vi "Dispose Report.vi"(0 "report in":refnum<class "NI_Word.lvclass">, 5 "wait until printing completed? (T)":bool=TRUE, 9 "save changes? (F)":bool, 11 "error in (no error)":errorcluster, 12 "close report? (T)":bool=TRUE) -> (15 "error out":errorcluster)   [LabVIEW 2015, in "NI_Word.lvclass"]
doc: "Closes the report and releases its interface, which saves memory."
uses:
  <vilib>/Utility/NIReport.llb/Word/NI_Word.lvclass
  <vilib>/Utility/NIReport.llb/Word/NI_Word.lvclass/NI_Word.ctl
  <vilib>/addons/_office/NI_ReportGenerationToolkit.lvlib
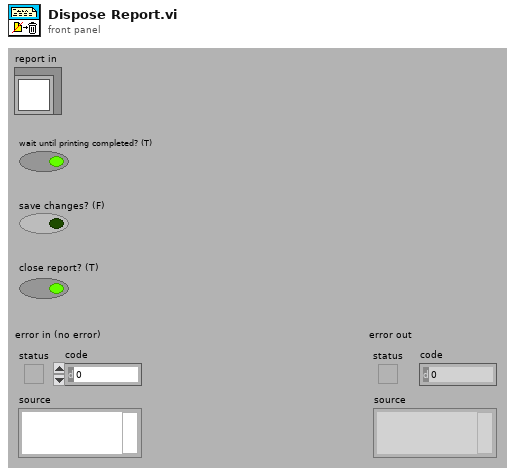
[diagram p1: front panel]
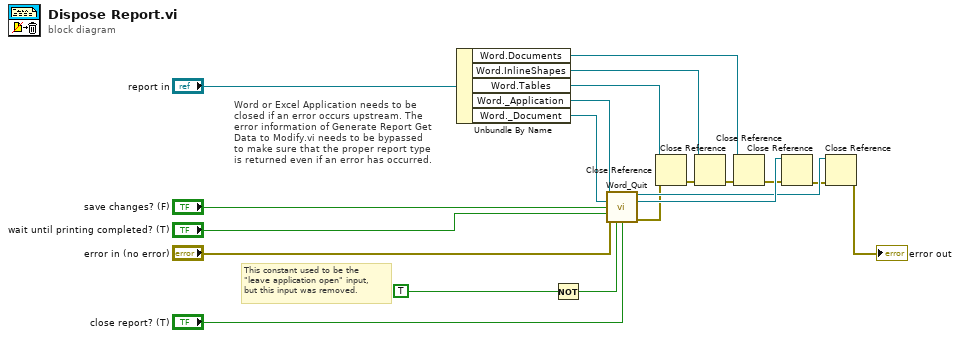
[diagram p0: block diagram]
diagram:
  # "This constant used to be the\n\"leave application open\" input,\nbut this input was removed."
  # "Word or Excel Application needs to be closed if an error occurs upstream. The error information of Generate Report Get Data to Modify.vi needs to be bypassed to make sure that the proper report type is returned even if an error has occurred."
  n1 = Unbundle By Name("report in") -> ("Word.Documents"=w13:refnum<k7>, "Word.InlineShapes"=w12:refnum<k7>, "Word.Tables"=w11:refnum<k7>, "Word._Application"=w17:refnum<k7>, "Word._Document"=w20:refnum<k7>)
  n2 = Not(x=TRUE) -> (.not. x?=w15:bool)
  n3 = call <vilib>:"Word_Quit.vi"("Word._Application in"=w17, "Word._Document in"=w20, "save changes?"="save changes? (F)", "wait until print completed?"="wait until printing completed? (T)", "error in(no error)"="error in (no error)", "Close Application"=w15, "Close Report"="close report? (T)") -> ("Word._Application out"=w18:refnum<k7>, "Word._Document out"=w19:refnum<k7>, "error out"=w16:errorcluster)  [unwired: 6 out]
  n4 = Close Reference(reference=w11, error in (no error)=w16) -> (error out=w9:errorcluster)
  n5 = Close Reference(reference=w12, error in (no error)=w9) -> (error out=w10:errorcluster)
  n6 = Close Reference(reference=w13, error in (no error)=w10) -> (error out=w8:errorcluster)
  n7 = Close Reference(reference=w19, error in (no error)=w8) -> (error out=w14:errorcluster)
  n8 = Close Reference(reference=w18, error in (no error)=w14) -> (error out=→"error out":errorcluster)
